vi "TrajectoryGenerate_Make_Quintic_CtrlVect.vi"(8 "traj_config":T7 {"End Velocity" format="%20.4f"; "StartVelocity" format="%20.4f"; "Max Acceleration" format="%20.4f"; "MaxVelocity" format="%20.4f"}, 11 "input_ControlVectors":T1[](array[typedef])) -> (0 "error out":errorcluster, 3 "TRAJECTORY":T2 {"States"."POSE"."ROTATION"."SIN" format="%13.4f"; "States"."POSE"."ROTATION"."COS" format="%13.4f"; "States"."POSE"."ROTATION"."VALUE" format="%13.4f"; "States"."POSE"."TRANSLATION"."Y" format="%14.3f"; "States"."POSE"."TRANSLATION"."X" format="%14.3f"; "TotalTImeSecs" format="%20.3f"})   [LabVIEW 2019, in "Trajectory_Library.lvlib"]
doc: "Generates a trajectory from the given quintic control vectors and config. This method uses quintic hermite splines -- therefore, all points must be represented by control vectors. Continuous curvature is guaranteed in this method.\n\nParameters:\n - ControlVectors - Array of quintic control vectors.\n - Trajectory Config - The configuration for the trajectory.\n\nReturns:\n - Trajectory -- Created trajectory data structure\n - Error Out - Returned error cluster"
uses:
  Trajectory_Library.lvlib
  TypeDef/ROTATION2D.ctl
  TypeDef/TRANSLATION2D.ctl
  TypeDef/POSEwCURVATURE.ctl
  TypeDef/POSE2D.ctl
  TypeDef/TRAJ_STATE.ctl
  TypeDef/TRAJECTORY.ctl
  TypeDef/TRAJ_CONFIG.ctl
  TypeDef/SPLINE_CTRL_VECTOR.ctl
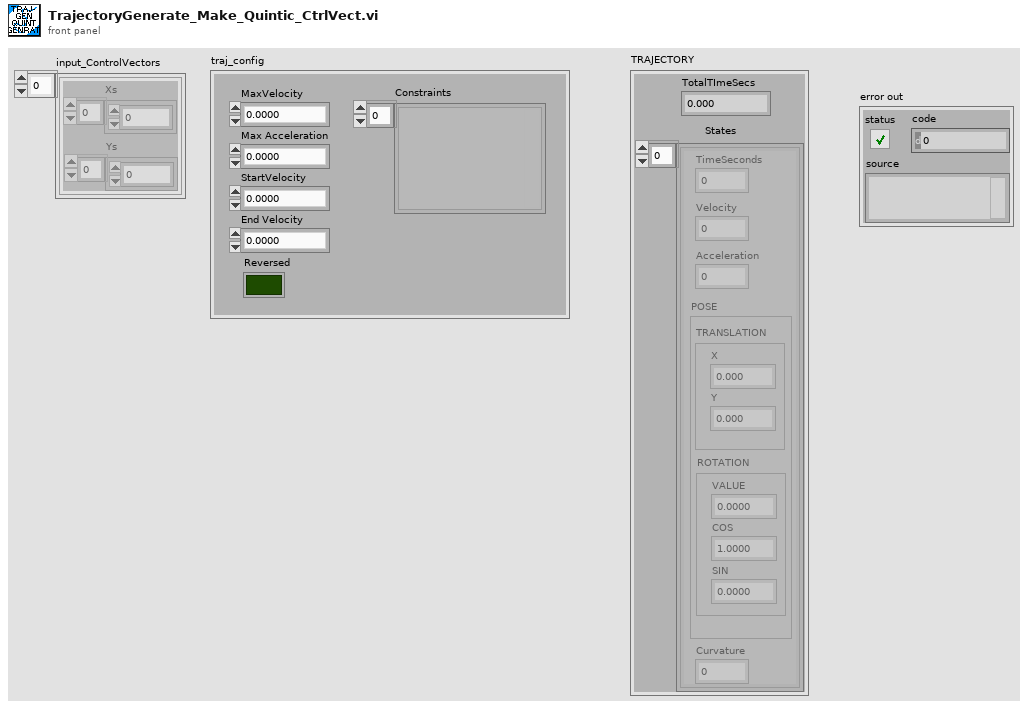
[diagram p1: front panel]
types:
  T1 = typedef "Trajectory_Library.lvlib/SPLINE_CTRL_VECTOR.ctl" = cluster{"Xs":dbl[], "Ys":dbl[]}
  T2 = typedef "Trajectory_Library.lvlib/TRAJECTORY.ctl" = cluster{"TotalTImeSecs":dbl, "States":T3[]}
  T3 = typedef "Trajectory_Library.lvlib/TRAJ_STATE.ctl" = cluster{"TimeSeconds":dbl, "Velocity":dbl, "Acceleration":dbl, "POSE":T4, "Curvature":dbl}
  T4 = typedef "Trajectory_Library.lvlib/POSE2D.ctl" = cluster{"TRANSLATION":T5, "ROTATION":T6}
  T5 = typedef "Trajectory_Library.lvlib/TRANSLATION2D.ctl" = cluster{"X":dbl, "Y":dbl}
  T6 = typedef "Trajectory_Library.lvlib/ROTATION2D.ctl" = cluster{"VALUE":dbl, "COS":dbl, "SIN":dbl}
  T7 = typedef "Trajectory_Library.lvlib/TRAJ_CONFIG.ctl" = cluster{"MaxVelocity":dbl, "Max Acceleration":dbl, "StartVelocity":dbl, "End Velocity":dbl, "Reversed":bool, "Constraints":variant[]}
  T8 = typedef "Trajectory_Library.lvlib/SPLINE.ctl" = cluster{"Degree":i32, "Coefficients":T9}
  T9 = typedef "NI_Matrix.lvlib/RealMatrix.ctl" = dbl[][]
  T10 = typedef "Trajectory_Library.lvlib/POSEwCURVATURE.ctl" = cluster{"CURVATURE":dbl, "POSE":T4}
  T11 = typedef "WPILib_Math.lvlib/TRANSLATION2D.ctl" = cluster{"X":dbl, "Y":dbl}
  T12 = typedef "WPILib_Math.lvlib/TRANSFORM2D.ctl" = cluster{"TRANSLATION":T11, "ROTATION":T13, "xF":bool}
  T13 = typedef "WPILib_Math.lvlib/ROTATION2D.ctl" = cluster{"VALUE":dbl, "COS":dbl, "SIN":dbl}
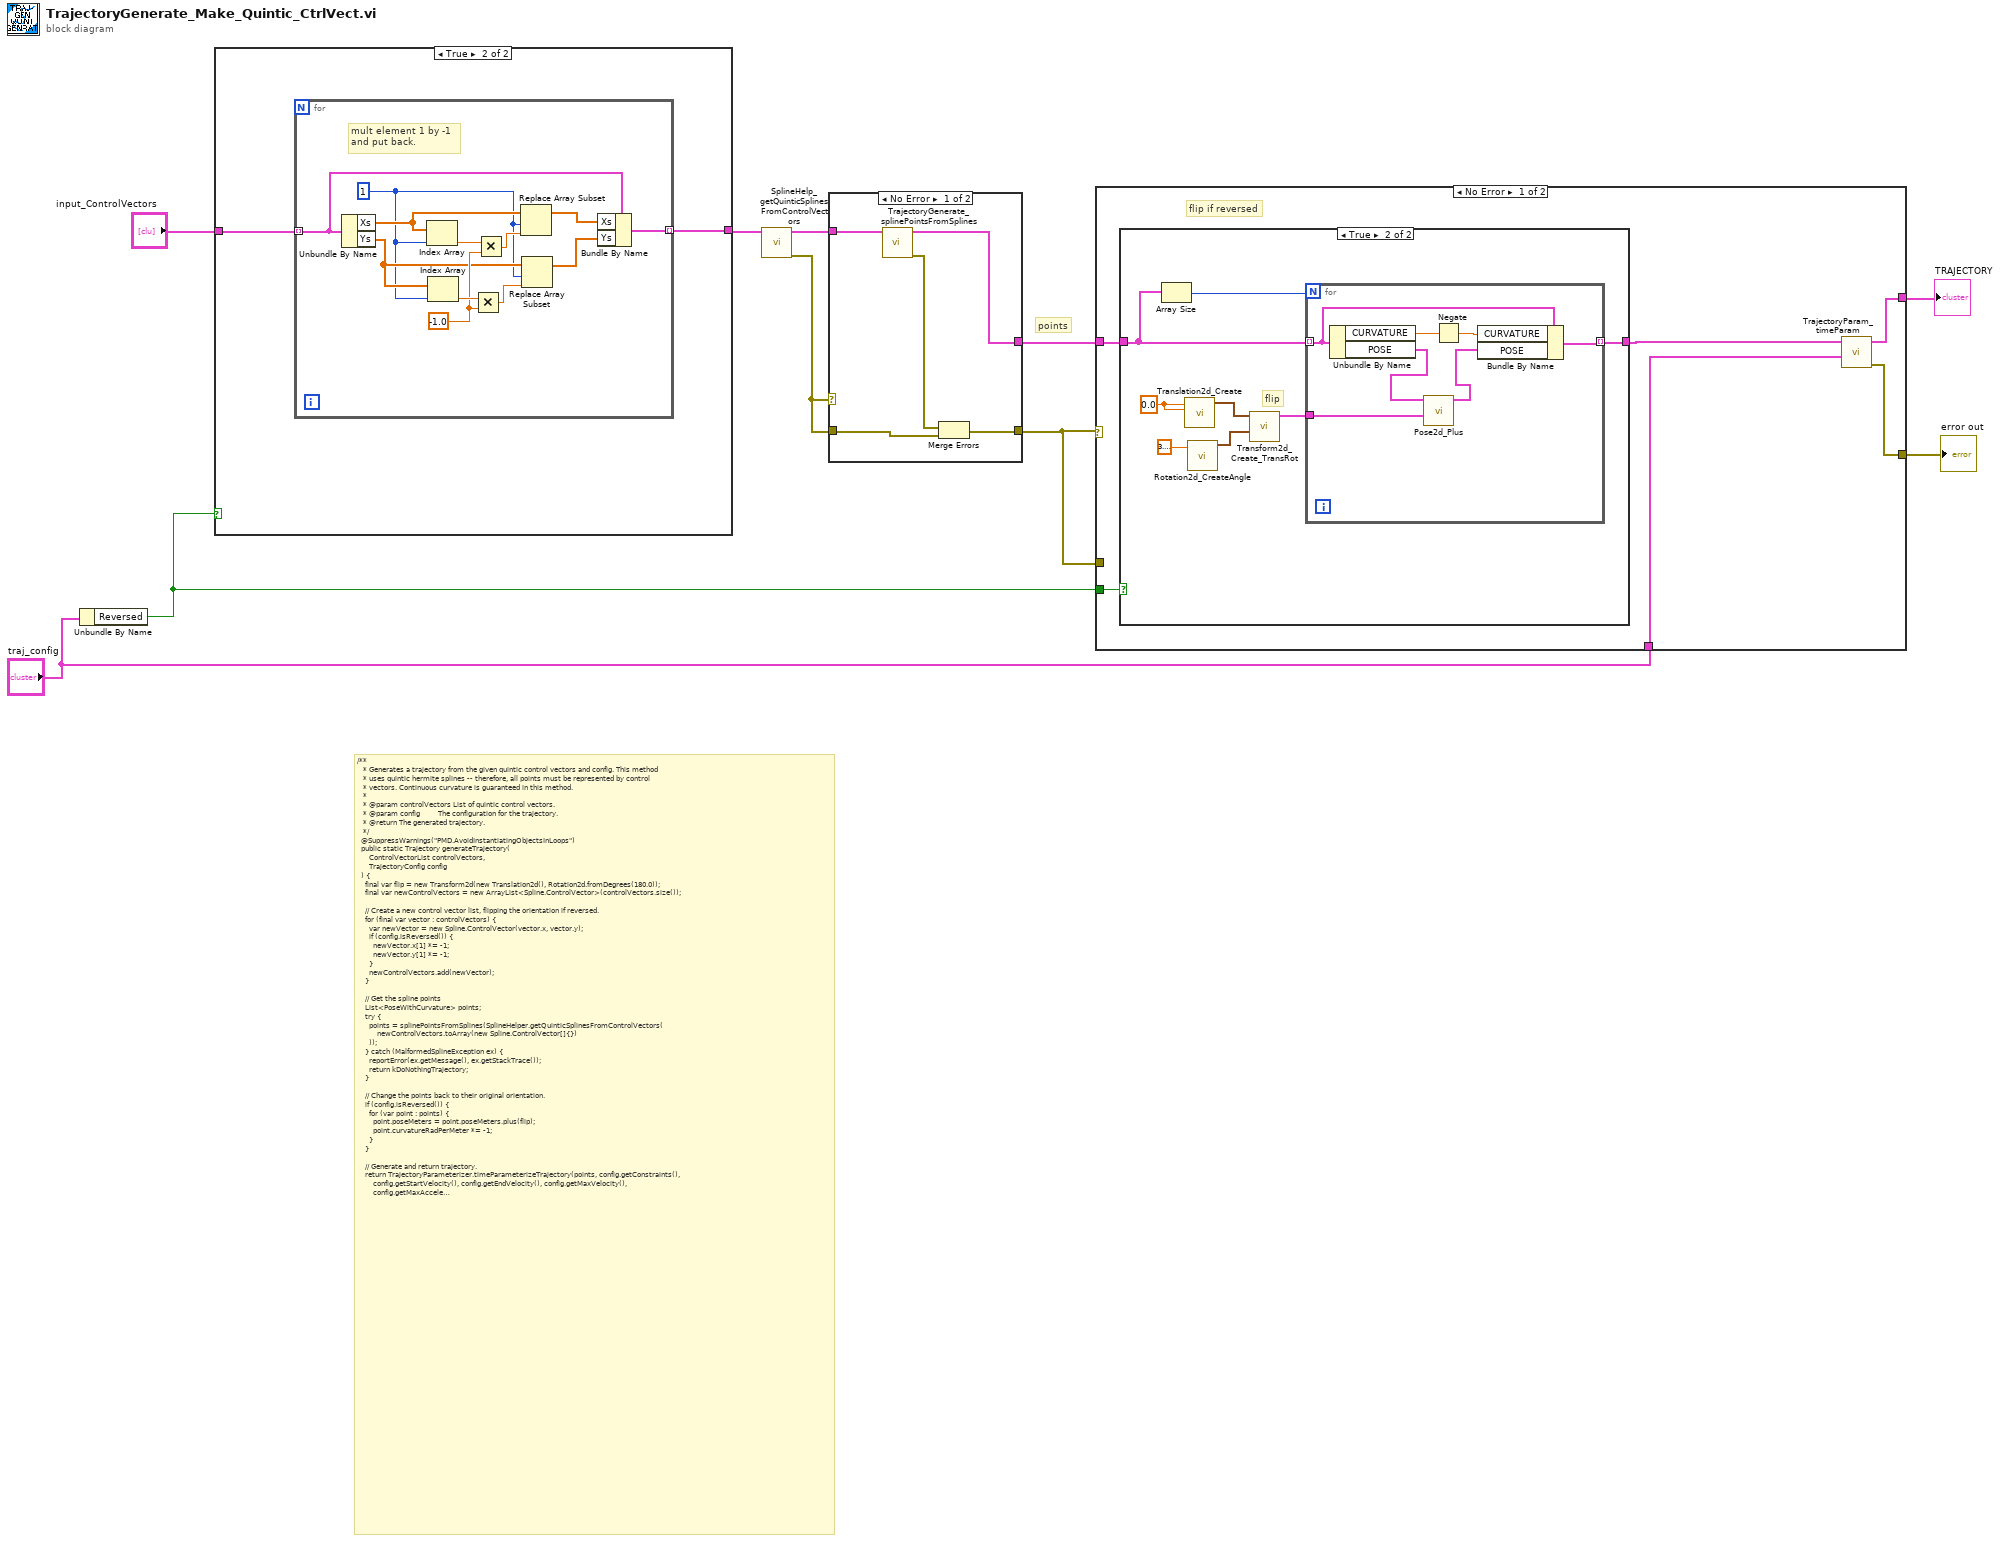
[diagram p0: block diagram]
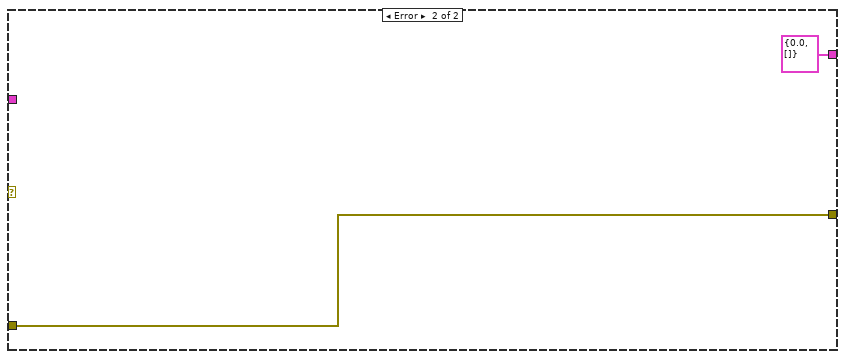
[diagram p3: hidden frame]
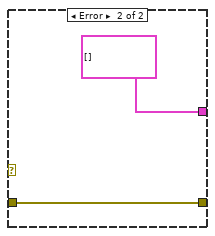
[diagram p4: hidden frame]
diagram:
  # "/**\n   * Generates a trajectory from the given quintic control vectors and config. This method\n   * uses quintic hermite splines -- therefore, all points must be represented by control\n   * vectors. Continuous curvature is guaranteed in this method.\n   *\n   * @param controlVectors List of quintic control vectors.\n   * @param config         The configuration for the trajectory.\n   * @return The generated trajectory.\n   */\n  @SuppressWarnings(\"PMD.AvoidInstantiatingObjectsInLoops\")\n  public static Trajectory generateTrajectory(\n      ControlVectorList controlVectors,\n      TrajectoryConfig config\n  ) {\n    final var flip = new Transform2d(new Translation2d(), Rotation2d.fromDegrees(180.0));\n    final var newControlVectors = new ArrayList<Spline.ControlVector>(controlVectors.size());\n\n    // Create a new control vector list, flipping the orientation if reversed.\n    for (final var vector : controlVectors) {\n      var newVector = new Spline.ControlVector(vector.x, vector.y);\n      if (config.isReversed()) {\n        newVector.x[1] *= -1;\n        newVector.y[1] *= -1;\n      }\n      newControlVectors.add(newVector);\n    }\n\n    // Get the spline points\n    List<PoseWithCurvature> points;\n    try {\n      points = splinePointsFromSplines(SplineHelper.getQuinticSplinesFromControlVectors(\n          newControlVectors.toArray(new Spline.ControlVector[]{})\n      ));\n    } catch (MalformedSplineException ex) {\n      reportError(ex.getMessage(), ex.getStackTrace());\n      return kDoNothingTrajectory;\n    }\n\n    // Change the points back to their original orientation.\n    if (config.isReversed()) {\n      for (var point : points) {\n        point.poseMeters = point.poseMeters.plus(flip);\n        point.curvatureRadPerMeter *= -1;\n      }\n    }\n\n    // Generate and return trajectory.\n    return TrajectoryParameterizer.timeParameterizeTrajectory(points, config.getConstraints(),\n        config.getStartVelocity(), config.getEndVelocity(), config.getMaxVelocity(),\n        config.getMaxAcceleration(), config.isReversed());\n\n  }"
  # "points"
  n1 = Unbundle By Name("traj_config") -> ("Reversed"=w7:bool)
  n2 = case shown="True" w7 {
    tunnel: "input_ControlVectors" -> [w11 w13]
    tunnel: [w11 w12] -> w10
    frame False {
    }
    frame True {
      n3 = for {
        tunnel: w13 -> [w17] mode=indexing
        tunnel: [w14] -> w12 mode=indexing
        w24 = -1.0
        w19 = 1 ("index")
        # "mult element 1 by -1\nand put back."
        n4 = Unbundle By Name(w17) -> ("Xs"=w22:dbl[], "Ys"=w20:dbl[])
        n5 = Index Array(array=w22, index=w19) -> (element=w23:dbl)
        n6 = Index Array(array=w20, index=w19) -> (element=w25:dbl)
        n7 = Multiply(x=w25, y=w24) -> (x*y=w18:dbl)
        n8 = Multiply(x=w23, y=w24) -> (x*y=w21:dbl)
        n9 = Replace Array Subset(array=w22, new element=w21, index=w19) -> (w16:dbl[])
        n10 = Replace Array Subset(array=w20, new element=w18, index=w19) -> (w15:dbl[])
        n11 = Bundle By Name(cluster=w17, "Xs"=w16, "Ys"=w15) -> (w14:T1)
      }
    }
  }
  n12 = call "SplineHelp_getQuinticSplinesFromControlVectors.vi"("ControlVectors"=w10) -> ("error out"=w9:errorcluster, "splines"=w5:T8[])  [unwired: 9 in]
  n13 = case shown="No Error" w9 {
    tunnel: [w30 w32] -> w6
    tunnel: w9 -> [w29 w32]
    tunnel: w5 -> [w27 _]
    tunnel: [w28 T10[] [] ("ArrayPoseWithCurvature")] -> w4
    frame No Error {
      n14 = call "TrajectoryGenerate_splinePointsFromSplines.vi"("inputSPLINE"=w27) -> ("error out"=w26:errorcluster, "ArrayPoseWithCurvature"=w28:T10[])  [unwired: 9 in]
      n15 = Merge Errors(w26, w29) -> (w30:errorcluster)
    }
    frame Error {
    }
  }
  n16 = case shown="No Error" w6 {
    tunnel: w6 -> [_ w56]
    tunnel: [w34 w56] -> w8
    tunnel: w7 -> [w38 _]
    tunnel: w4 -> [w37 _]
    tunnel: [w35 T2 {"TotalTImeSecs"=0.0, "States"=[]} ("TRAJECTORY")] -> w3
    tunnel: "traj_config" -> [w33 _]
    frame No Error {
      # "flip if reversed"
      n17 = case shown="True" w38 {
        tunnel: w37 -> [w39 w46]
        tunnel: [w39 w45] -> w36
        frame False {
        }
        frame True {
          w41 = 0.0 ("X")
          # "flip"
          n18 = Array Size(array=w46) -> (size(s)=w47:i32)
          n19 = call "Translation2d_Create.vi"("Y"=w41, "X"=w41) -> ("TRANSLATION"=w43:T11)  [unwired: 9 in]
          n20 = call "Rotation2d_CreateAngle.vi"("Angle"=3.141592653589793) -> ("ROTATION"=w44:T6)  [unwired: 10 in]
          n21 = call "Transform2d_Create_TransRot.vi"("ROTATION"=w44, "TRANSLATION"=w43) -> ("TRANSFORM"=w40:T12)  [unwired: 9 in]
          n22 = for {
            N: w47 -> [_]
            tunnel: w46 -> [w53] mode=indexing
            tunnel: [w52] -> w45 mode=indexing
            tunnel: w40 -> [w50]
            n23 = Unbundle By Name(w53) -> ("CURVATURE"=w54:dbl, "POSE"=w49:T4)
            n24 = call "Pose2d_Plus.vi"("other TRANSFORM"=w50, "in POSE"=w49) -> ("out POSE"=w48:T4)  [unwired: 9 in]
            n25 = Negate(x=w54) -> (-x=w51:dbl)
            n26 = Bundle By Name(cluster=w53, "CURVATURE"=w51, "POSE"=w48) -> (w52:T10)
          }
        }
      }
      n27 = call "TrajectoryParam_timeParam.vi"("TRAJECTORY_CONFIG"=w33, "points"=w36) -> ("error out"=w34:errorcluster, "TRAJECTORY"=w35:T2)  [unwired: 8 in]
    }
    frame Error {
    }
  }
  "TRAJECTORY" <- w3
  "error out" <- w8
